vi "Write User Event (Array).vi"(6 "優先度（通常）":T1, 7 "EvCmd[]":string[](array[string]), 8 "エラー入力（エラーなし）":errorcluster, 10 "データ[]":variant[](array[variant]), 11 "ユーザイベント入力":refnum<user-event>) -> (0 "エラー出力":errorcluster, 3 "ユーザイベント出力":refnum<user-event>)   [LabVIEW 2016]
uses:
  <vilib>/event_ctls.llb/usereventprio.ctl
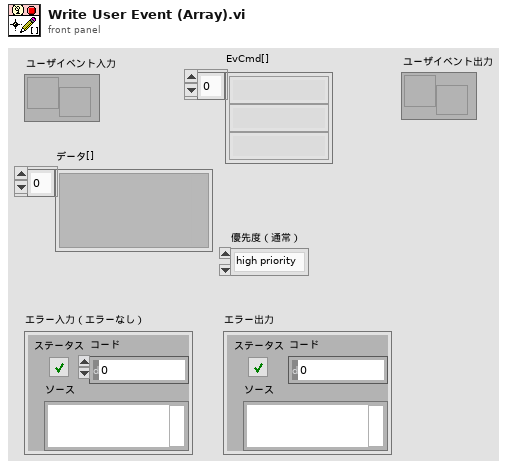
[diagram p1: front panel]
types:
  T1 = typedef "usereventprio.ctl" = enum32{"high priority", "normal priority"}
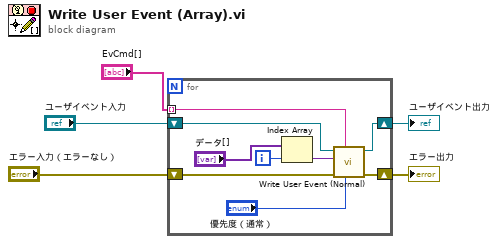
[diagram p0: block diagram]
diagram:
  n1 = for {
    shift-right: [w9] -> w4
    shift-left: "エラー入力（エラーなし）" -> [w10]
    tunnel: "EvCmd[]" -> [w12] mode=indexing
    shift-right: [w8] -> w1
    shift-left: "ユーザイベント入力" -> [w11]
    i -> [w13]
    n2 = Index Array(array="データ[]", index=w13) -> (element=w6:variant)
    n3 = call "Write User Event (Normal).vi"("優先度（通常）"="優先度（通常）", "EvCmd"=w12, "エラー入力（エラーなし）"=w10, "データ"=w6, "ユーザイベント入力"=w11) -> ("エラー出力"=w9:errorcluster, "ユーザイベント出力"=w8:refnum<user-event>)  [unwired: 5 in]
  }
  "エラー出力" <- w4
  "ユーザイベント出力" <- w1
